vi "VGI Read Datas.vi"(8 "error in (no error)":errorcluster, 9 "PinMask":u16, 10 "DevIndex":i32, 11 "DevType":i32) -> (0 "error out":errorcluster, 2 "function return":i32, 3 "pData":u16)   [LabVIEW 2012, in "ControlGPIO.lvlib"]
doc: "int WINAPI VGI_ReadDatas(int DevType,int DevIndex,unsigned short PinMask,unsigned short *pData);"
uses:
  ControlGPIO.lvlib
  Ginkgo_Driver.dll
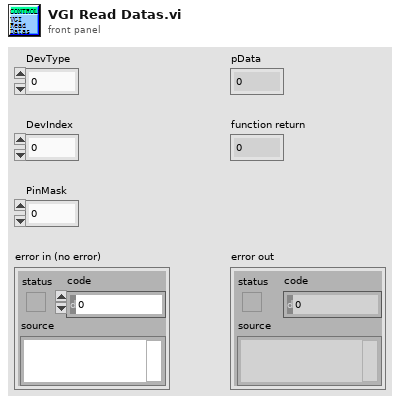
[diagram p1: front panel]
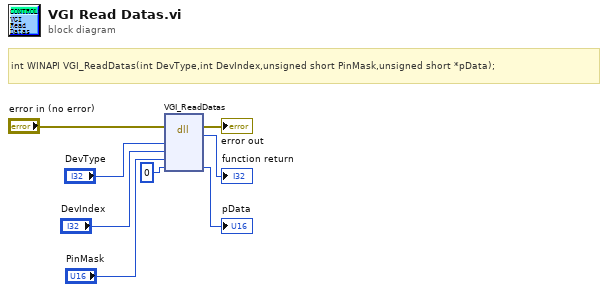
[diagram p0: block diagram]
diagram:
  # "int WINAPI VGI_ReadDatas(int DevType,int DevIndex,unsigned short PinMask,unsigned short *pData);"
  n1 = dll-call lib="E:/Project/vt_ginkgo/truck/Ginkgo Driver/vs2010/Ginkgo_USB-I2C_API_v2.0.3.0/lib/labview_32bit/ControlGPIO/Ginkgo_Driver.*" fn="VGI_ReadDatas"(error in="error in (no error)", "DevType"="DevType", "DevIndex"="DevIndex", "PinMask"="PinMask", "pData"=u16 0) -> (error out=→"error out":errorcluster, →"function return":i32, "pData"=→"pData":u16)  [unwired: 5 in, 1 out]
